vi "RGB_Img_sub.vi"(1 "pixel size":i32=10, 2 "B_2D(28x28)":i32[][](array[numeric]), 3 "G_2D(28x28)":i32[][](array[numeric]), 4 "R_2D(28x28)":i32[][](array[numeric])) -> (0 "picture":picture)   [LabVIEW 2021]
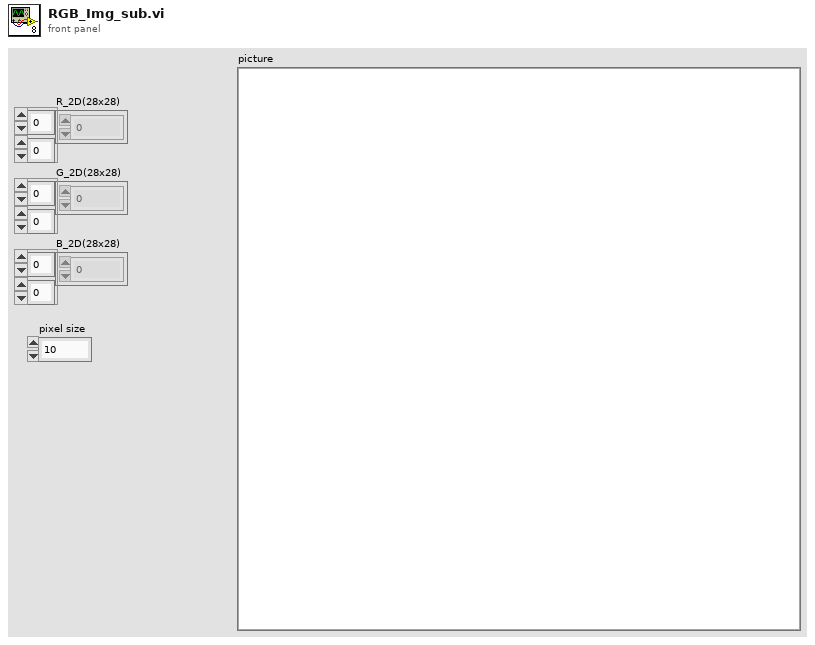
[diagram p1: front panel]
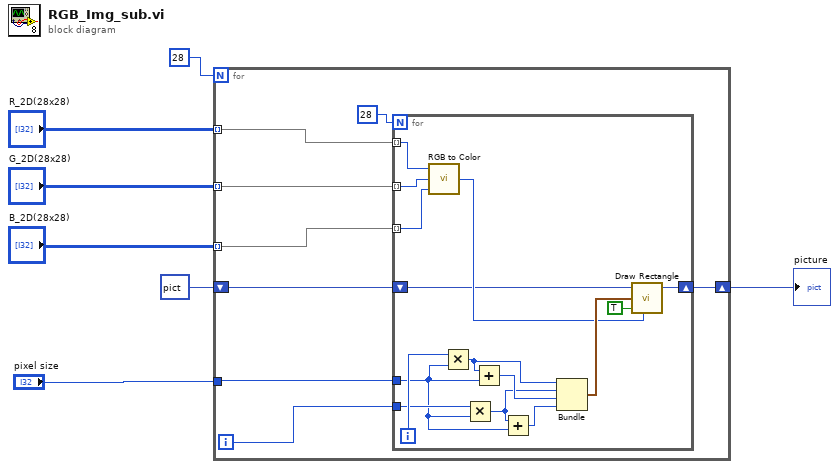
[diagram p0: block diagram]
diagram:
  n1 = for {
    N: 28 -> [_]
    tunnel: "R_2D(28x28)" -> [w15] mode=indexing
    tunnel: "G_2D(28x28)" -> [w14] mode=indexing
    tunnel: "B_2D(28x28)" -> [w13] mode=indexing
    tunnel: "pixel size" -> [w11]
    shift-right: [w9] -> w4
    shift-left: picture data[5B] ("picture") -> [w10]
    i -> [w12]
    n2 = for {
      N: 28 -> [_]
      tunnel: w15 -> [w29] mode=indexing
      tunnel: w14 -> [w28] mode=indexing
      tunnel: w13 -> [w27] mode=indexing
      tunnel: w12 -> [w21]
      tunnel: w11 -> [w20]
      shift-right: [w16] -> w9
      shift-left: w10 -> [w17]
      i -> [w22]
      n3 = call <vilib>:"RGB to Color.vi"("B"=w27, "G"=w28, "R"=w29) -> ("Color"=w18:u32)
      n4 = Multiply(x=w22, y=w20) -> (x*y=w26:i32)
      n5 = Multiply(x=w21, y=w20) -> (x*y=w24:i32)
      n6 = Add(x=w26, y=w20) -> (x+y=w25:i32)
      n7 = Add(x=w24, y=w20) -> (x+y=w23:i32)
      n8 = Bundle(w26, w24, w25, w23) -> (w19:cluster{i32, i32, i32, i32})  [unwired: 1 in]
      n9 = call <vilib>:"Draw Rectangle.vi"("picture"=w17, "rect"=w19, "fill?(F)"=TRUE, "color(black)"=w18) -> ("new picture"=w16:picture)  [unwired: 5 in]
    }
  }
  "picture" <- w4
